vi "Set Releys Test.vi"() -> ()   [LabVIEW 2023, in "DO_Relay.lvlib"]
uses:
  DO_Relay.lvlib
  <userlib>/DAQNavi Polymorphic VI/create/DAQNavi Create Channel(DI-Digital Input).vi
  <userlib>/DAQNavi Polymorphic VI/create/DAQNavi Create Channel(DO-Digital Output).vi
  <userlib>/DAQNavi Polymorphic VI/write/DAQNavi Write (Digtial 1D U8 NChan 1Samp).vi
  <userlib>/DAQNavi Polymorphic VI/read/DAQNavi Read (Digital 1D Wfm NChan 1Samp).vi
  <userlib>/DAQNavi Polymorphic VI/read/DAQNavi Read (Digital 1D U8 1Chan NSamp).vi
panel:
  out "data 3":digitalwaveform[](array[waveform])
  out "data 2":digitalwaveform(waveform)={"t0"=timestamp(0 s since 1904-01-01), "dt"=1.0, "Y"={"transitions"=[], "data"=[]}}
  out "Digital Waveform Graph":digitalwaveform[](graph)
  out "data":u8
  out "number":u32
  out "Boolean array":bool[](array[boolean])
  in  "binary array":u8[](array[numeric])
  out "read back data":u8[](array[numeric])
  out "physical channels":string="DemoDevice,BID#0/port0:1" caption="property value"
  out "number of samples written per channel":u32
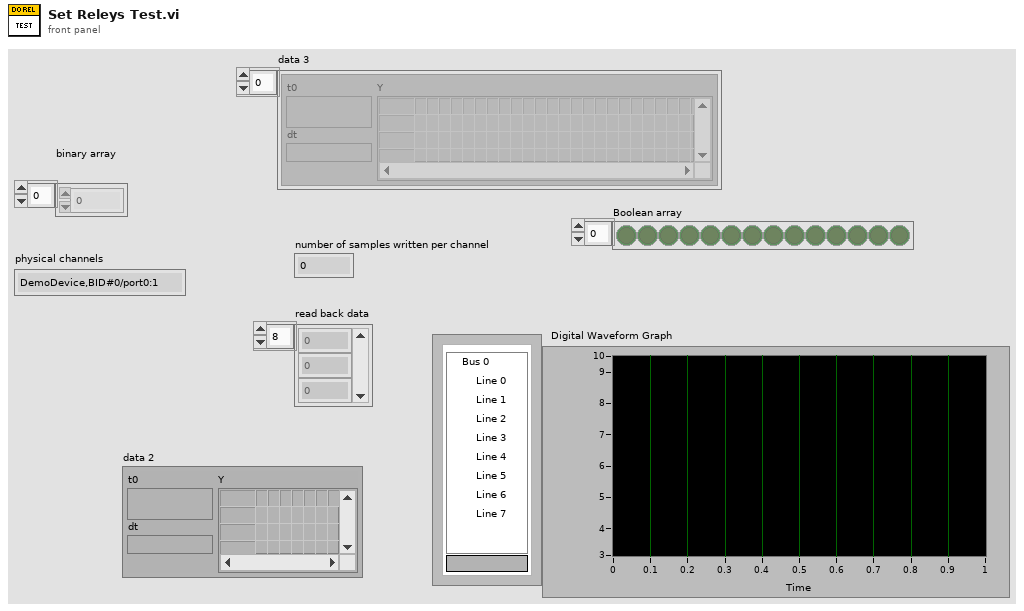
[diagram p1: front panel]
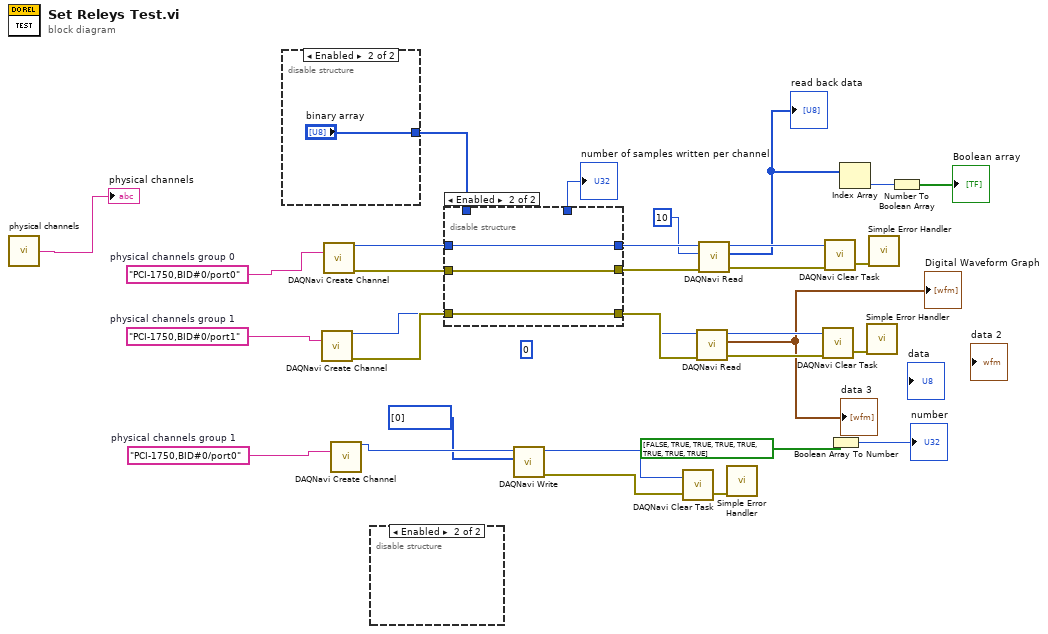
[diagram p0: block diagram]
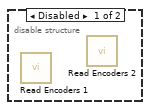
[diagram p2: hidden frame]
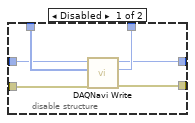
[diagram p3: hidden frame]
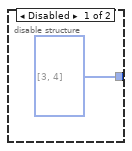
[diagram p4: hidden frame]
diagram:
  w8 = "PCI-1750,BID#0/port0"  # physical channels group 1
  (unwired) 0 ("portBit")
  w10 = "PCI-1750,BID#0/port1"  # physical channels group 1
  w9 = "PCI-1750,BID#0/port0"  # physical channels group 0
  n1 = call "physical channels"() -> ("property value"=→"physical channels":string)  [unwired: 1 out]
  n2 = disable-structure shown="Enabled" {
    disable-tunnel: [u8[] [3, 4] ("binary array") "binary array"] -> w30
    frame Disabled {
    }
    frame Enabled {
    }
  }
  n3 = call-poly <userlib>:"DAQNavi Create Channel.vi"("physical channels"=w10) -> ("task out"=w12:i32, "error out"=w13:errorcluster)  [unwired: 4 in, 9 out]
  n4 = call-poly <userlib>:"DAQNavi Create Channel.vi"("physical channels"=w9) -> ("task out"=w29:i32, "error out"=w28:errorcluster)  [unwired: 4 in, 9 out]
  n5 = call-poly <userlib>:"DAQNavi Create Channel.vi"("physical channels"=w8) -> ("task out"=w7:i32)  [unwired: 4 in, 10 out]
  n6 = disable-structure shown="Enabled" {
    frame Disabled {
      n7 = call "Read Encoders 1.vi"() -> ()  [unwired: 10 in, 2 out]
      n8 = call "Read Encoders 2.vi"() -> ()  [unwired: 8 in, 4 out]
    }
    frame Enabled {
    }
  }
  n9 = disable-structure shown="Enabled" {
    disable-tunnel: [w40 _] -> w31
    disable-tunnel: w30 -> [w39 _]
    disable-tunnel: w29 -> [w38 w44]
    disable-tunnel: w28 -> [w37 w43]
    disable-tunnel: [w36 w44] -> w27
    disable-tunnel: [w35 w43] -> w26
    disable-tunnel: w12 -> [_ w41]
    disable-tunnel: w13 -> [_ w42]
    disable-tunnel: [_ w41] -> w14
    disable-tunnel: [_ w42] -> w15
    frame Disabled {
      n10 = call-poly <userlib>:"DAQNavi Write.vi"("error in (no error)"=w37, "data"=w39, "task in"=w38) -> ("error out"=w35:errorcluster, "number of samples written per channel"=w40:u32, "task out"=w36:i32)  [unwired: 1 in, 5 out]
    }
    frame Enabled {
    }
  }
  "number of samples written per channel" <- w31
  n11 = call-poly <userlib>:"DAQNavi Write.vi"("data"=u8[] [0], "task in"=w7) -> ("error out"=w3:errorcluster, "task out"=w4:i32)  [unwired: 2 in, 6 out]
  n12 = call <userlib>:"DAQNavi Clear Task.vi"("error in (no error)"=w3, "task in"=w4) -> ("error out"=w5:errorcluster)  [unwired: 1 out]
  n13 = call-poly <userlib>:"DAQNavi Read.vi"("error in (no error)"=w15, "task in"=w14) -> ("error out"=w17:errorcluster, "data"=→"Digital Waveform Graph" →"data 3":digitalwaveform[], "task out"=w16:i32)  [unwired: 1 in, 6 out]
  n14 = call-poly <userlib>:"DAQNavi Read.vi"("error in (no error)"=w26, "number of samples per channel to read"=u32 10, "task in"=w27) -> ("error out"=w24:errorcluster, "data"=w22:u8[], "task out"=w25:i32)  [unwired: 1 in, 5 out]
  "read back data" <- w22
  n15 = call <vilib>:"Simple Error Handler.vi"("error in (no error)"=w5) -> ()  [unwired: 2 in, 7 out]
  n16 = call <userlib>:"DAQNavi Clear Task.vi"("error in (no error)"=w17, "task in"=w16) -> ("error out"=w11:errorcluster)  [unwired: 1 out]
  n17 = call <userlib>:"DAQNavi Clear Task.vi"("error in (no error)"=w24, "task in"=w25) -> ("error out"=w32:errorcluster)  [unwired: 1 out]
  n18 = Boolean Array To Number(Boolean array=bool[] [FALSE, TRUE, TRUE, TRUE, TRUE, TRUE, TRUE, TRUE] ("Boolean array 2")) -> (number=→"number":u32)
  n19 = Index Array(array=w22) -> (element=w21:u8)  [unwired: 1 in]
  n20 = call <vilib>:"Simple Error Handler.vi"("error in (no error)"=w11) -> ()  [unwired: 2 in, 7 out]
  n21 = call <vilib>:"Simple Error Handler.vi"("error in (no error)"=w32) -> ()  [unwired: 2 in, 7 out]
  n22 = Number To Boolean Array(number=w21) -> (Boolean array=→"Boolean array":bool[])
